vi "criteria_initialize.vi"(8 "error in (no error)":errorcluster, 10 "recipe_data":variant, 11 "criteria":variant) -> (0 "error out":errorcluster)   [LabVIEW 2015, in "example_01.lvlib"]
uses:
  example_01.lvlib
  _controls/recipes.ctl
  <userlib>/antonio-alexander/lv-recipe-machine/lv-recipe-machine.lvlib
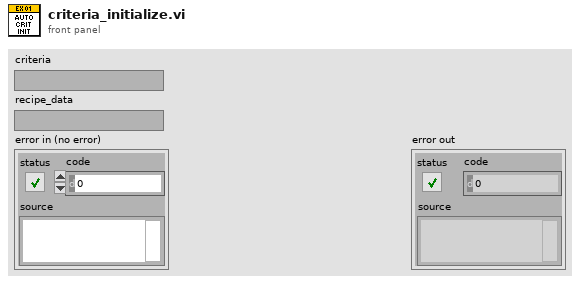
[diagram p1: front panel]
types:
  T1 = typedef "example_01.lvlib/recipes.ctl" = enum16{"<recipes>", "wait_random", "random_wait", "count", "comparison", "launch", "<null>"}
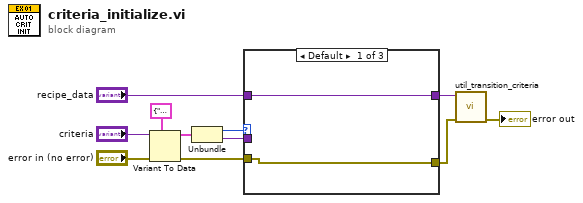
[diagram p0: block diagram]
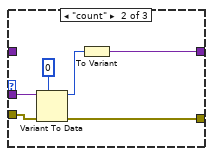
[diagram p2: hidden frame]
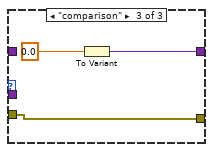
[diagram p3: hidden frame]
diagram:
  n1 = Variant To Data(error in="error in (no error)", type=cluster{"recipe":T1, variant} {"recipe"=enum."<recipes>", variant}, Variant="criteria") -> (data=w7:cluster{"recipe":T1, variant}, error out=w4:errorcluster)
  n2 = Unbundle(w7) -> ("recipe"=w6:T1, w5:variant)
  n3 = case shown="Default" w6 {
    tunnel: w5 -> [_ w14 _]
    tunnel: w4 -> [w12 w19 w20]
    tunnel: "recipe_data" -> [w13 _ _]
    tunnel: [w13 w16 w22] -> w2
    tunnel: [w12 w15 w20] -> w1
    frame Default {
    }
    frame "count" {
      n4 = Variant To Data(error in=w19, type=0, Variant=w14) -> (data=w17:i32, error out=w15:errorcluster)
      n5 = To Variant(anything=w17) -> (Variant=w16:variant)
    }
    frame "comparison" {
      n6 = To Variant(anything=0.0) -> (Variant=w22:variant)
    }
  }
  n7 = call <userlib>:"util_transition_criteria.vi"("error in (no error)"=w1, "recipe_data"=w2) -> ("error out"=→"error out":errorcluster)  [unwired: 9 in]
